vi "triangle test.vi"(5 "Boolean 2":bool, 9 "Boolean 3":bool) -> (8 "Boolean":bool)   [LabVIEW 2018]
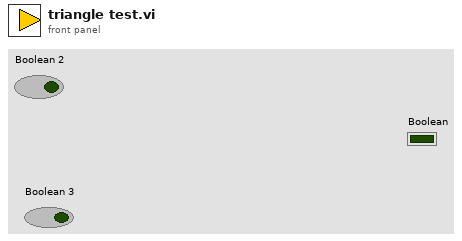
[diagram p1: front panel]
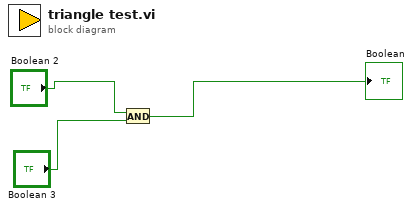
[diagram p0: block diagram]
diagram:
  n1 = And(x="Boolean 2", y="Boolean 3") -> (x .and. y?=→"Boolean":bool)
